vi "Build Tool.vi"(1 "Tool Buttons":T1) -> (0 "Tool":refnum<class "Tool.lvclass">)   [LabVIEW 2020, in "Map Model.lvlib" / "Map Model.lvclass"]
uses:
  Map Model.lvclass
  Type Definitions/Tool Buttons.ctl
  Tools/Tool/Tool.lvclass
  Tools/Pan/Pan.lvclass
  E:/Project/Labview-Projects/Completed projects/Map Editor/Models/Map Model/Tools/Tool/Tool.lvclass
  Tools/Pencil/Pencil.lvclass
  Tools/Line/Line.lvclass
  Tools/Eraser/Eraser.lvclass
  Tools/Rectangle Select/Rectangle Select.lvclass
  Tools/Deselect/Deselect.lvclass
  Tools/Crop/Crop.lvclass
  Tools/Rotate/Rotate.lvclass
  Tools/Set Origin/Set Origin.lvclass
  Tools/Zoom In/Zoom In.lvclass
  Tools/Zoom Out/Zoom Out.lvclass
panel:
  # "NOTICE -- YOU MUST LEAVE THIS NOTICE IN PLACE.\n\nCopyright (c) 2017, LIANG LIU Shawn.Liu.cn@gmail.com\nAll rights reserved.\n\nRedistribution and use in source and binary forms, with or without modification, are permitted provided that the following conditions are met:\n-Redistributions of source code must retain the above copyright notice, this list of conditions and the following disclaimer.\n-Redistributions in binary form must reproduce the above copyright notice, this list of conditions and the following disclaimer in the documentation and/or other materials provided with the distribution.\n-Neither the name of the eLp nor the names of its contributors may be used to endorse or promote products derived from this software without specific prior written permission.\n\nTHIS SOFTWARE IS PROVIDED BY THE COPYRIGHT HOLDERS AND CONTRIBUTORS \"AS IS\" AND ANY EXPRESS OR IMPLIED WARRANTIES, INCLUDING, BUT NOT LIMITED TO, THE IMPLIED WARRANTIES OF MERCHANTABILITY AND FITNESS FOR A PARTICULAR PURPOSE ARE DISCLAIMED. IN NO EVENT SHALL THE COPYRIGHT HOLDER OR CONTRIBUTORS BE LIABLE FOR ANY DIRECT, INDIRECT, INCIDENTAL, SPECIAL, EXEMPLARY, OR CONSEQUENTIAL DAMAGES (INCLUDING, BUT NOT LIMITED TO, PROCUREMENT OF SUBSTITUTE GOODS OR SERVICES; LOSS OF USE, DATA, OR PROFITS; OR BUSINESS INTERRUPTION) HOWEVER CAUSED AND ON ANY THEORY OF LIABILITY, WHETHER IN CONTRACT, STRICT LIABILITY, OR TORT (INCLUDING NEGLIGENCE OR OTHERWISE) ARISING IN ANY WAY OUT OF THE USE OF THIS SOFTWARE, EVEN IF ADVISED OF THE POSSIBILITY OF SUCH DAMAGE."
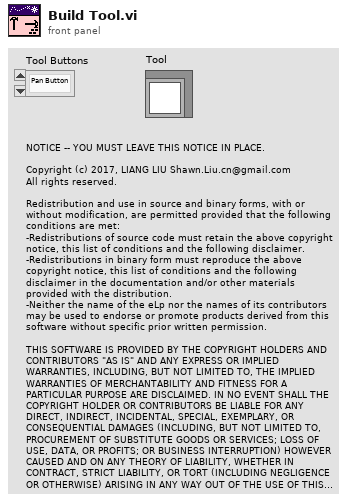
[diagram p1: front panel]
types:
  T1 = typedef "Tool Buttons.ctl" = enum32{"Pan Button", "Pencil Button", "Line Button", "Eraser Button", "Rectangle Select Button", "Deselect Button", "Crop Button", "Rotate Button", "Set Origin Button", "Zoom In Button", "Zoom Out Button"}
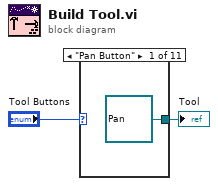
[diagram p0: block diagram]
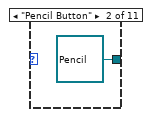
[diagram p2: hidden frame]
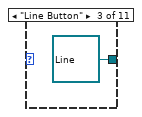
[diagram p3: hidden frame]
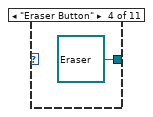
[diagram p4: hidden frame]
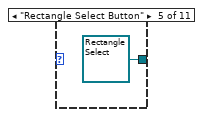
[diagram p5: hidden frame]
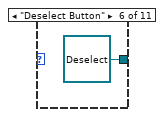
[diagram p6: hidden frame]
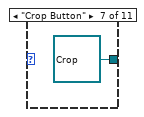
[diagram p7: hidden frame]
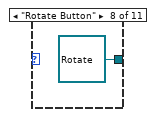
[diagram p8: hidden frame]
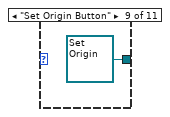
[diagram p9: hidden frame]
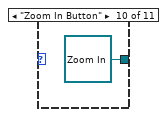
[diagram p10: hidden frame]
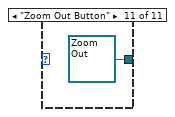
[diagram p11: hidden frame]
diagram:
  n1 = case shown="\"Pan Button\"" "Tool Buttons" {
    tunnel: [refnum<class "Pan.lvclass"> refnum ("Map Model.lvlib:Pan.lvclass") refnum<class "Pencil.lvclass"> refnum ("Map Model.lvlib:Pencil.lvclass") refnum<class "Line.lvclass"> refnum ("Map Model.lvlib:Line.lvclass") refnum<class "Eraser.lvclass"> refnum ("Map Model.lvlib:Eraser.lvclass") refnum<class "Rectangle Select.lvclass"> refnum ("Map Model.lvlib:Rectangle Select.lvclass") refnum<class "Deselect.lvclass"> refnum ("Map Model.lvlib:Deselect.lvclass") refnum<class "Crop.lvclass"> refnum ("Map Model.lvlib:Crop.lvclass") refnum<class "Rotate.lvclass"> refnum ("Map Model.lvlib:Rotate.lvclass") refnum<class "Set Origin.lvclass"> refnum ("Map Model.lvlib:Set Origin.lvclass") refnum<class "Zoom In.lvclass"> refnum ("Map Model.lvlib:Zoom In.lvclass") refnum<class "Zoom Out.lvclass"> refnum ("Map Model.lvlib:Zoom Out.lvclass")] -> w1
    frame "Pan Button" {
    }
    frame "Pencil Button" {
    }
    frame "Line Button" {
    }
    frame "Eraser Button" {
    }
    frame "Rectangle Select Button" {
    }
    frame "Deselect Button" {
    }
    frame "Crop Button" {
    }
    frame "Rotate Button" {
    }
    frame "Set Origin Button" {
    }
    frame "Zoom In Button" {
    }
    frame "Zoom Out Button" {
    }
  }
  "Tool" <- w1
